vi "Read Watershed Image.vi"(8 "error in (no error)":errorcluster, 11 "Video Cam Processor in":refnum<class "Video Cam Processor.lvclass">) -> (0 "error out":errorcluster, 2 "Image":T1, 3 "Video Cam Processor out":refnum<class "Video Cam Processor.lvclass">)   [LabVIEW 2018, in "Video Cam Processor.lvclass"]
uses:
  Video Cam Processor.lvclass
  <vilib>/vision/Image Controls.llb/IMAQ Image.ctl
  Video Cam Processor.lvclass/Video Cam Processor.ctl
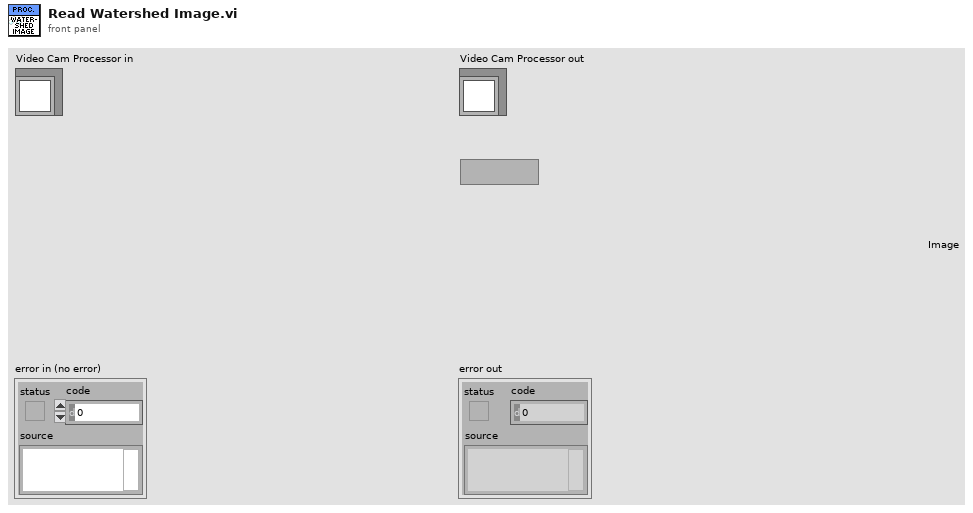
[diagram p1: front panel]
types:
  T1 = typedef "IMAQ Image.ctl" = refnum<image>
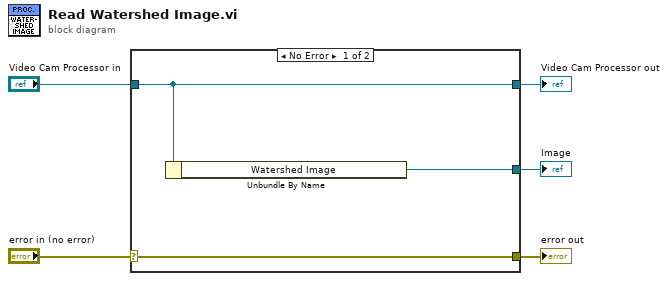
[diagram p0: block diagram]
diagram:
  n1 = case shown="No Error" "error in (no error)" {
    selector: "error in (no error)" -> [w8 w9]
    tunnel: [w8 w9] -> w4
    tunnel: [w7 w10] -> w2
    tunnel: "Video Cam Processor in" -> [w7 w10]
    tunnel: [w6 _] -> w1
    frame No Error {
      n2 = Unbundle By Name(w7) -> ("Watershed Image"=w6:T1)
    }
    frame Error {
    }
  }
  "error out" <- w4
  "Video Cam Processor out" <- w2
  "Image" <- w1
